vi "ModbusTestMasterHmi.vi"() -> ()   [LabVIEW 2018, in "ModbusTestMasterHmi.lvlib"]
uses:
  ModbusTestMasterHmi.lvlib
  <vilib>/Platform/TimedLoop/XDataNode/timing_clust.ctl
  <vilib>/Platform/TimedLoop/XDataNode/nitl_modes.ctl
  <vilib>/Platform/TimedLoop/XDataNode/wakeup.ctl
  <vilib>/platform/TimedLoop/XDataNode/XDataNode.xnode
  <vilib>/Platform/TimedLoop/XDataNode/XDNodeRunTimeDep.lvlib
panel:
  out "Input Registry Float #2":sgl
  out "Input Registry Float #1":sgl
  in  "Holding Registry Float #2":sgl(slide) scale=0.0..10.0
  in  "Holding Registry Float #1":sgl(slide) scale=0.0..10.0
  in  "Update Rate":dbl(slide) scale=0.0..10.0
  out "Input Registry 32 #2":i32(knob) scale=-500000.0..500000.0
  out "Input Registry 32 #1":i32(knob) scale=-500000.0..500000.0
  in  "Holding Registry 32 #2":i32(knob) scale=-1000000.0..1000000.0
  in  "Holding Registry 32 #1":i32(knob) scale=-1000000.0..1000000.0
  in  "Update":bool
  out "Updating":bool
  out "Off Hook":bool
  out "Communication Failure":bool
  in  "Stop":bool
  out "Cycle":i32
  in  "Frequency":dbl(slide) scale=0.0..10.0
  out "Discrete Input 10001":bool
  in  "Coil 00002":bool
  in  "Coil 00001":bool
  out "Discrete Input 10002":bool
  in  "Holding Registry 40002":i16(slide) min=0 max=255 step=1 scale=0.0..255.0
  in  "Holding Registry 40001":i16(slide) min=0 max=255 step=1 scale=0.0..255.0
  out "Input Registry 30002":dbl(slide) scale=0.0..1024.0
  out "Input Registry 30001":dbl(slide) scale=0.0..1024.0
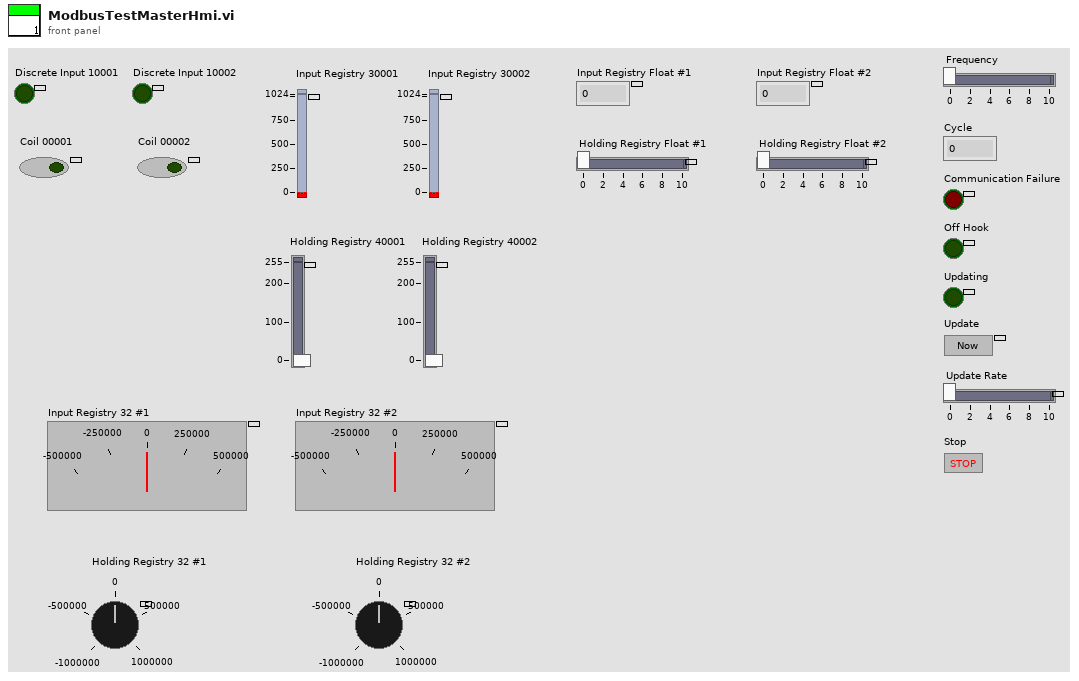
[diagram p1: front panel]
types:
  T1 = typedef "XDNodeRunTimeDep.lvlib/timing_clust.ctl" = cluster{"Expected End [f-1]":u64, "Actual End [f-1]":u64, "Finished Late? [f-1]":bool, "Expected End [i-1]":u64, "Actual End [i-1]":u64, "Finished Late? [i-1]":bool, "Expected Start [i]":u64, "Actual Start [i]":u64, "Expected Start [f]":u64, "Actual Start [f]":u64, "Source Name":string, "Structure Name":string, "Period":i64, "Deadline":i64, "Offset":i64, "Start":i64, "Priority":i32, "Timeout":i32, "Mode":T2, "Wakeup Reason":T3, "Error":errorcluster, "Source Type":string, "Secondary Source Type":string, "Global End Time":u64, "Global Start Time":u64, "Frame Duration":u64, "Iteration Duration":u64, "Assigned CPU":i32, "I/O Scan Engine Mode":u32}
  T2 = typedef "XDNodeRunTimeDep.lvlib/nitl_modes.ctl" = enum32{"No Change", "Process missed periods, maintain original phase", "Discard missed periods, maintain original phase", "Process missed periods, ignore original phase", "Discard missed periods, ignore original phase"}
  T3 = typedef "XDNodeRunTimeDep.lvlib/wakeup.ctl" = enum32{"Normal", "Aborted", "Asynchronous wakeup", "Timing source error", "Timed loop error", "Timeout"}
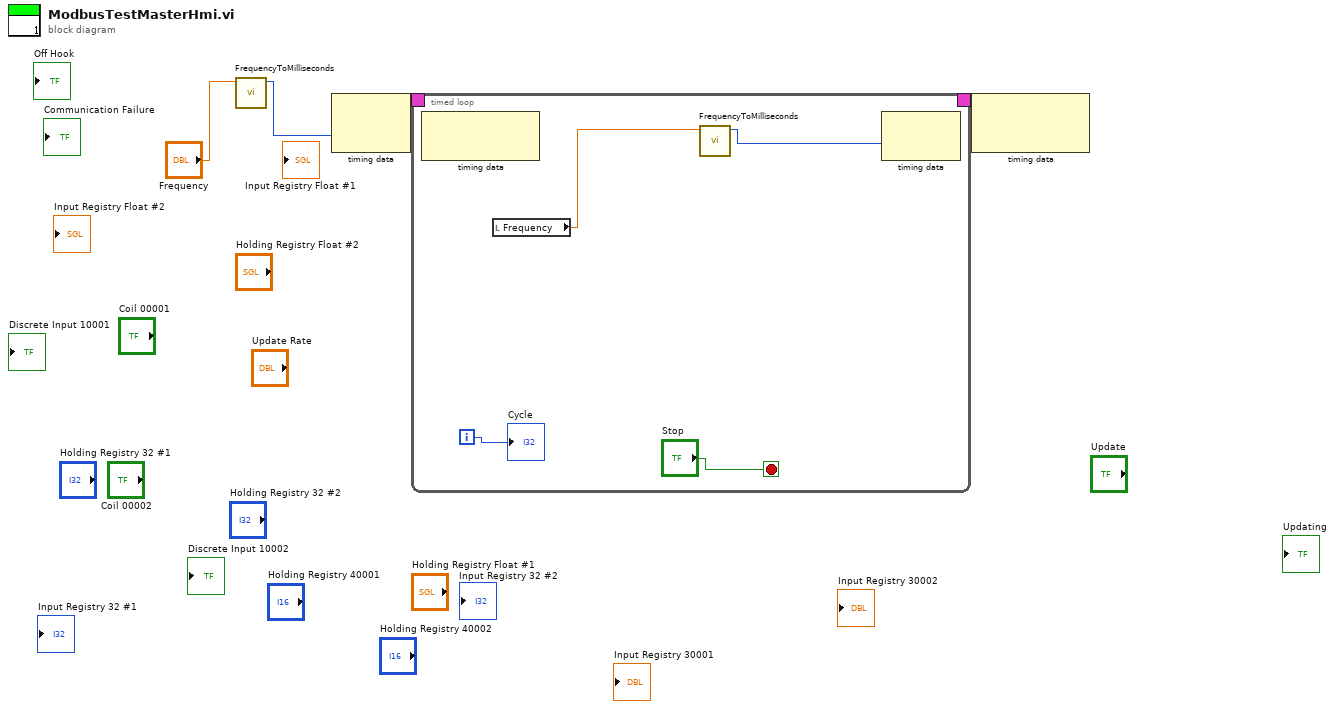
[diagram p0: block diagram]
diagram:
  n1 = call "FrequencyToMilliseconds.vi"("Frequency"="Frequency") -> ("Numeric"=w1:i64)  [unwired: 10 in]
  n2 = node-c288(w1) -> (w4:T1)  [unwired: 1 in]
  n3 = timed-loop {
    timing: w4 -> [_]
    timing-out: [_] -> w3
    i -> [w7]
    stop <- "Stop" stop-if-true
    n4 = node-c288() -> ()  [unwired: 1 in, 2 out]
    n5 = local read "Frequency"() -> (w5:dbl)
    n6 = call "FrequencyToMilliseconds.vi"("Frequency"=w5) -> ("Numeric"=w6:i64)  [unwired: 10 in]
    n7 = node-c288(w6) -> ()  [unwired: 1 in, 1 out]
    "Cycle" <- w7
  }
  n8 = node-c288(w3) -> ()  [unwired: 2 out]
